vi "Create All Message Queues Ascan.vi"(8 "error in (no error)":cluster{"状态":bool, "代码":i32, "源":string} caption="错误输入（无错误）") -> (0 "error out":cluster{"状态":bool, "代码":i32, "源":string} caption="错误输出", 3 "消息队列":T1)   [LabVIEW 2015, in "Message Queue.lvlib"]
doc: "本VI用于创建应用程序所需的所有消息队列。如应用程序需要两个以上消息队列，可右键单击上面的“消息队列”常量并选择打开自定义类型，将新的消息队列添加至该自定义类型，然后通过本VI进行初始化。"
uses:
  Message Queue.lvlib
  All Message Queues Ascan.ctl
  Message Cluster.ctl
  Enqueue Message (Single).vi
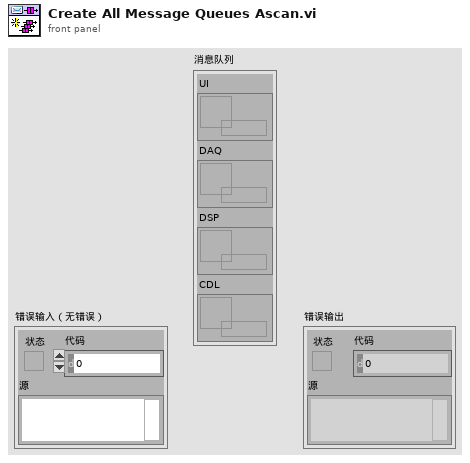
[diagram p1: front panel]
types:
  T1 = typedef "Message Queue.lvlib/All Message Queues Ascan.ctl" = cluster{"UI":refnum<queue>, "DAQ":refnum<queue>, "DSP":refnum<queue>, "CDL":refnum<queue>}
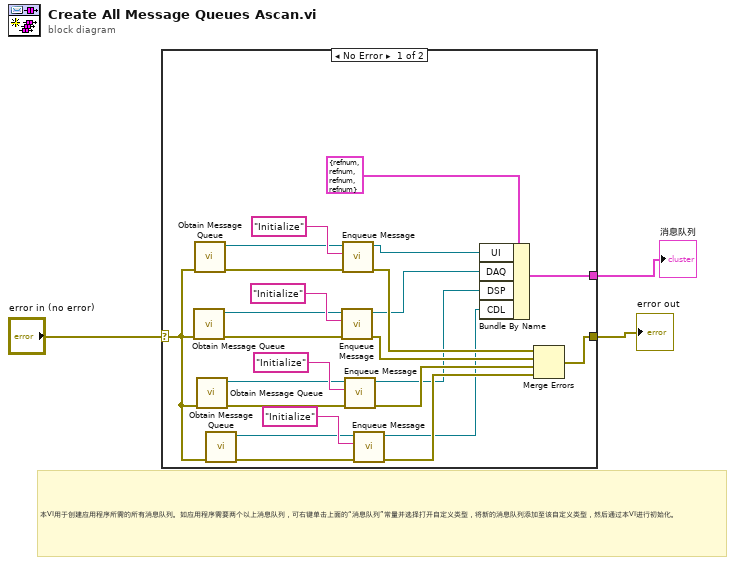
[diagram p0: block diagram]
diagram:
  # "本VI用于创建应用程序所需的所有消息队列。如应用程序需要两个以上消息队列，可右键单击上面的“消息队列”常量并选择打开自定义类型，将新的消息队列添加至该自定义类型，然后通过本VI进行初始化。"
  n1 = case shown="No Error" "error in (no error)" {
    selector: "error in (no error)" -> [w9 w28]
    tunnel: [w20 w28] -> w3
    tunnel: [w27 _] -> w1
    frame No Error {
      n2 = call "Obtain Message Queue.vi"("error in (no error)"=w9) -> ("error out"=w26:cluster{"状态":bool, "代码":i32, "源":string}, "消息队列"=w24:refnum<queue>)  [unwired: 9 in]
      n3 = call "Obtain Message Queue.vi"("error in (no error)"=w9) -> ("error out"=w12:cluster{"状态":bool, "代码":i32, "源":string}, "消息队列"=w10:refnum<queue>)  [unwired: 9 in]
      n4 = call "Obtain Message Queue.vi"("error in (no error)"=w9) -> ("error out"=w23:cluster{"状态":bool, "代码":i32, "源":string}, "消息队列"=w21:refnum<queue>)  [unwired: 9 in]
      n5 = call "Obtain Message Queue.vi"("error in (no error)"=w9) -> ("error out"=w17:cluster{"状态":bool, "代码":i32, "源":string}, "消息队列"=w15:refnum<queue>)  [unwired: 9 in]
      n6 = call-poly "Enqueue Message.vi"("error in (no error)"=w26, "消息"="Initialize" ("Message"), "消息队列"=w24) -> ("error out"=w19:cluster{"状态":bool, "代码":i32, "源":string}, "消息队列副本"=w6:refnum<queue>)  [unwired: 7 in]
      n7 = call-poly "Enqueue Message.vi"("error in (no error)"=w12, "消息"="Initialize" ("Message"), "消息队列"=w10) -> ("error out"=w8:cluster{"状态":bool, "代码":i32, "源":string}, "消息队列副本"=w7:refnum<queue>)  [unwired: 7 in]
      n8 = call-poly "Enqueue Message.vi"("error in (no error)"=w23, "消息"="Initialize" ("Message"), "消息队列"=w21) -> ("error out"=w18:cluster{"状态":bool, "代码":i32, "源":string}, "消息队列副本"=w5:refnum<queue>)  [unwired: 7 in]
      n9 = call-poly "Enqueue Message.vi"("error in (no error)"=w17, "消息"="Initialize" ("Message"), "消息队列"=w15) -> ("error out"=w14:cluster{"状态":bool, "代码":i32, "源":string}, "消息队列副本"=w4:refnum<queue>)  [unwired: 7 in]
      n10 = Bundle By Name(cluster=T1 {"UI"=refnum, "DAQ"=refnum, "DSP"=refnum, "CDL"=refnum} ("消息队列"), "UI"=w7, "DAQ"=w6, "DSP"=w5, "CDL"=w4) -> (w27:T1)
      n11 = Merge Errors(w8, w19, w18, w14) -> (w20:errorcluster)
    }
    frame Error {
    }
  }
  "error out" <- w3
  "消息队列" <- w1
